vi "Upgrade Refactor Data.vi"() -> (0 "refactor data":T1)   [LabVIEW 2020, in "MeasurementService Editor.lvlib"]
uses:
  MeasurementService Editor.lvlib
  Rename Refactor Data.ctl
  Rename Refactor Mapping Info.ctl
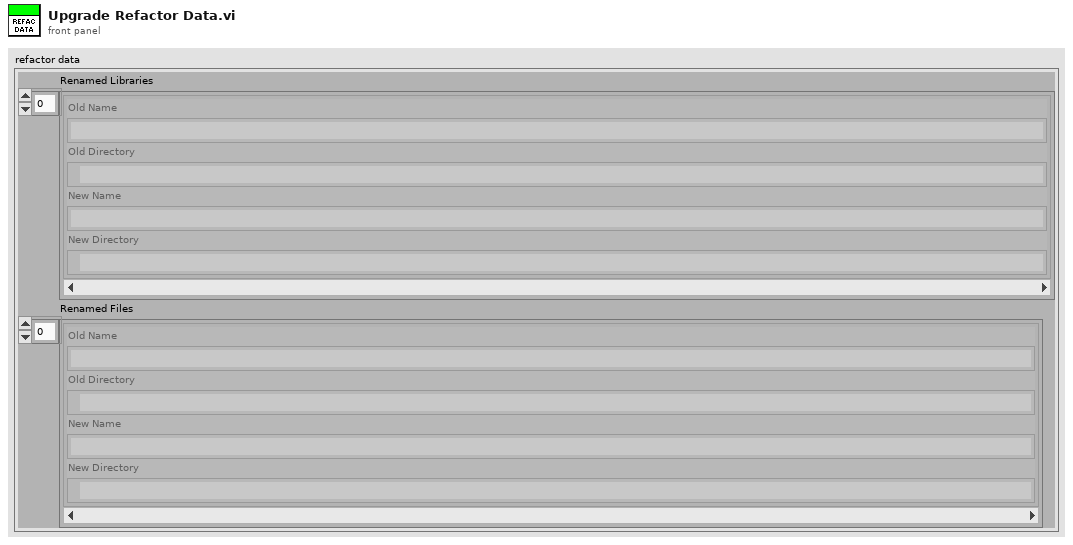
[diagram p1: front panel]
types:
  T1 = typedef "MeasurementService Editor.lvlib/Rename Refactor Data.ctl" = cluster{"Renamed Libraries":T2[], "Renamed Files":T2[]}
  T2 = typedef "MeasurementService Editor.lvlib/Rename Refactor Mapping Info.ctl" = cluster{"Old Name":string, "Old Directory":path, "New Name":string, "New Directory":path}
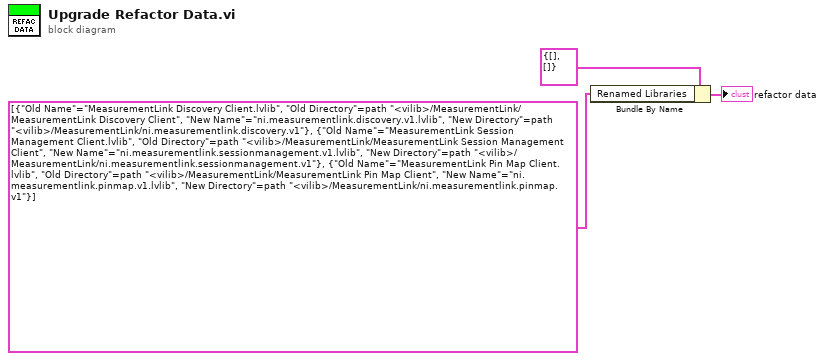
[diagram p0: block diagram]
diagram:
  n1 = Bundle By Name(cluster=T1 {"Renamed Libraries"=[], "Renamed Files"=[]} ("Rename Data"), "Renamed Libraries"=T2[] [{"Old Name"="MeasurementLink Discovery Client.lvlib", "Old Directory"=path "<vilib>/MeasurementLink/MeasurementLink Discovery Client", "New Name"="ni.measurementlink.discovery.v1.lvlib", "New Directory"=path "<vilib>/MeasurementLink/ni.measurementlink.discovery.v1"}, {"Old Name"="MeasurementLink Session Management Client.lvlib", "Old Directory"=path "<vilib>/MeasurementLink/MeasurementLink Session Management Client", "New Name"="ni.measurementlink.sessionmanagement.v1.lvlib", "New Directory"=path "<vilib>/MeasurementLink/ni.measurementlink.sessionmanagement.v1"}, {"Old Name"="MeasurementLink Pin Map Client.lvlib", "Old Directory"=path "<vilib>/MeasurementLink/MeasurementLink Pin Map Client", "New Name"="ni.measurementlink.pinmap.v1.lvlib", "New Directory"=path "<vilib>/MeasurementLink/ni.measurementlink.pinmap.v1"}]) -> (→"refactor data":T1)
